vi "Averaging Tool.vi"() -> ()   [LabVIEW 2009]
panel:
  in  "Tab Control":enum32{"Calculator", "Under the hood"}(tab)
  in  "Ratio and Error":dbl[][](array[numeric])
  out "Average":dbl
  out "Error":dbl
  out "% Error":dbl
  in  "Calculate":bool
  out "ratios":dbl[](array[numeric])
  out "errors":dbl[](array[numeric])
  out "First zero":i32
  # "Ratio"
  # "Error"
  # "If error is 0, that ratio and \nsubsequent ratios are left \nout of the calculation."
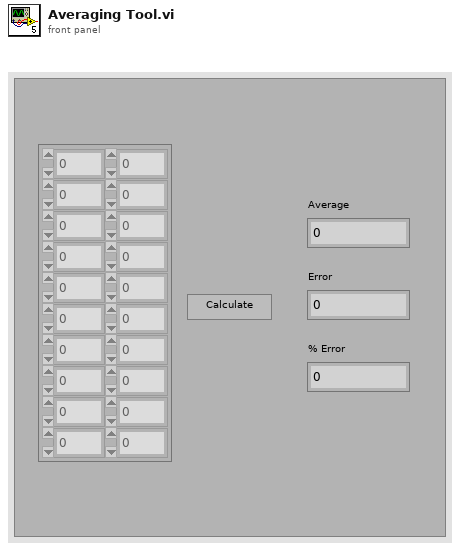
[diagram p1: front panel]
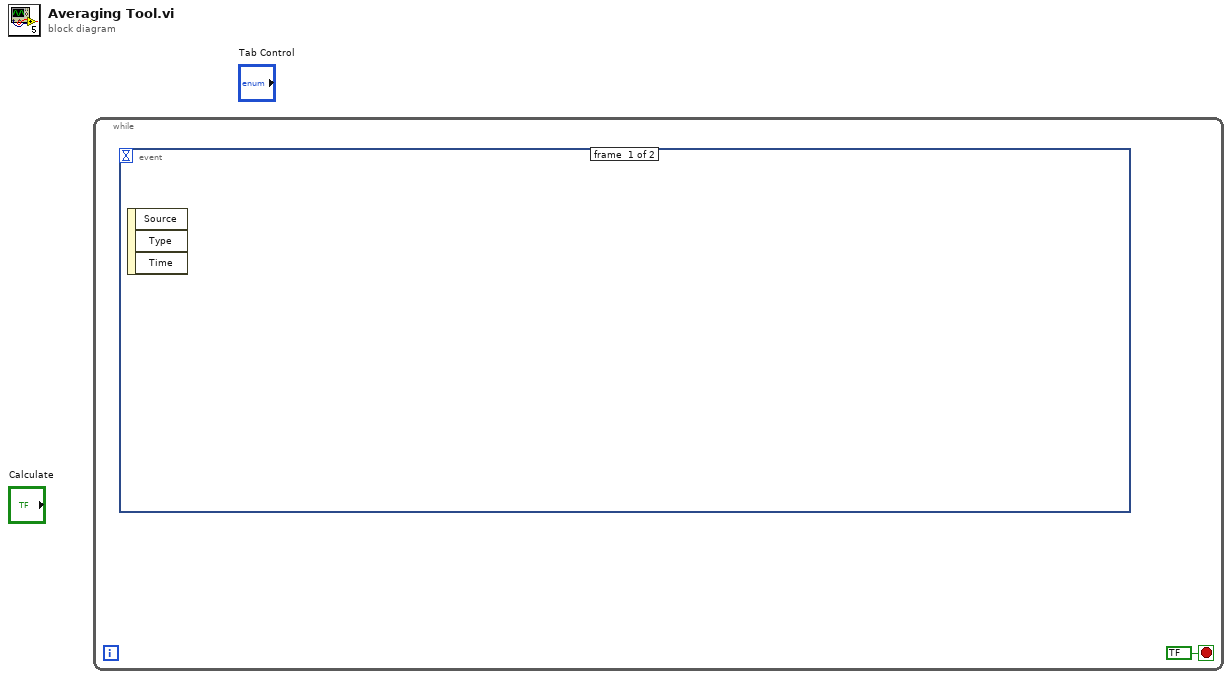
[diagram p0: block diagram]
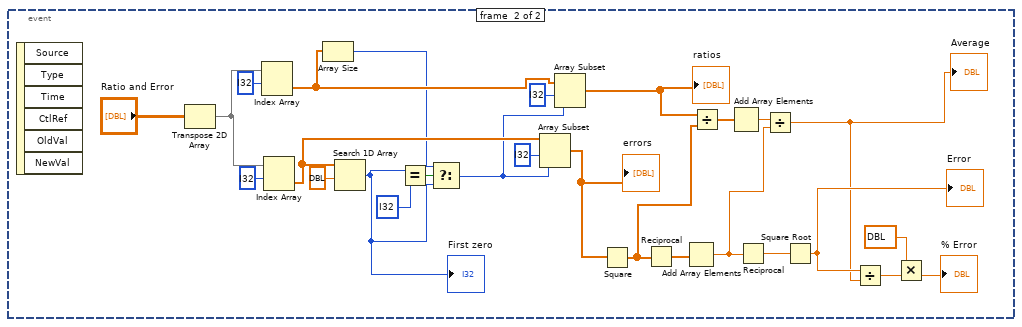
[diagram p2: hidden frame]
diagram:
  n1 = while {
    stop <- bool ? stop-if-true
    n2 = event shown="[1] \"Calculate\": Value Change" {
      selector: _ -> [_ _]
      dyn-events: _ -> [_ _]
      timeout: _ -> [_ _]
      event #0 {
        n3 = event-data() -> ()  [unwired: 1 in, 3 out]
      }
      event #1 {
        n4 = event-data() -> ()  [unwired: 1 in, 6 out]
        n5 = Transpose 2D Array(2D array="Ratio and Error") -> (transposed array=w25:dbl[][])
        n6 = Index Array(array=w25, index (row)=i32 ?) -> (element=w7:dbl[])  [unwired: 1 in]
        n7 = Index Array(array=w25, index (row)=i32 ?) -> (element=w14:dbl[])  [unwired: 1 in]
        n8 = Array Size(array=w7) -> (size(s)=w2:i32)
        n9 = Search 1D Array(1D array=w14, element=dbl ?) -> (index of element=w3:i32)  [unwired: 1 in]
        "First zero" <- w3
        n10 = Equal?(x=w3, y=i32 ? ("x")) -> (x = y?=w6:bool)
        n11 = Select(t=w2, s=w6, f=w3) -> (s? t:f=w5:i32)
        n12 = Array Subset(array=w14, index=i32 ?, length=w5) -> (w12:dbl[])
        "errors" <- w12
        n13 = Array Subset(array=w7, index=i32 ?, length=w5) -> (w10:dbl[])
        "ratios" <- w10
        n14 = Square(x=w12) -> (x^2=w22:dbl[])
        n15 = Reciprocal(x=w22) -> (1/x=w24:dbl[])
        n16 = Add Array Elements(numeric array=w24) -> (sum=w19:dbl)
        n17 = Divide(x=w10, y=w22) -> (x/y=w21:dbl[])
        n18 = Add Array Elements(numeric array=w21) -> (sum=w20:dbl)
        n19 = Reciprocal(x=w19) -> (1/x=w23:dbl)
        n20 = Divide(x=w20, y=w19) -> (x/y=w16:dbl)
        "Average" <- w16
        n21 = Square Root(x=w23) -> (sqrt(x)=w17:dbl)
        "Error" <- w17
        n22 = Divide(x=w17, y=w16) -> (x/y=w18:dbl)
        n23 = Multiply(x=dbl ?, y=w18) -> (x*y=→"% Error":dbl)
      }
    }
  }
